vi "json is equal.vi"(8 "error in (no error)":errorcluster, 9 "json string B":string, 10 "json string A":string, 11 "TestCase in":refnum<class "TestCase.lvclass">) -> (0 "error out":errorcluster, 3 "TestCase out":refnum<class "TestCase.lvclass">)   [LabVIEW 2017]
uses:
  <vilib>/addons/_JKI Toolkits/VI Tester/TestCase.llb/TestCase.lvclass
  <vilib>/National Instruments/Variant Data Manipulation/Path API/Read Value at Path(String).vi
  <vilib>/National Instruments/Variant JSON API/Variant JSON API.lvlib
  <vilib>/National Instruments/Variant Data Manipulation/Variant Data Manipulation.lvlib
  <vilib>/Utility/Data Type/NI_Data Type.lvlib
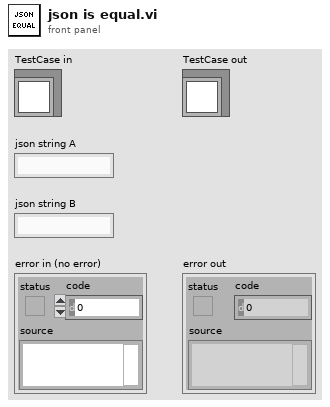
[diagram p1: front panel]
types:
  T1 = typedef "NI_Data Type.lvlib/Data Type.ctl" = enum8{"Invalid Type", "Void", "I8", "I16", "I32", "I64", "U8", "U16", "U32", "U64", "Single Float", "Double Float", "Extended Float", "Single Complex", "Double Complex", "Extended Complex", "Enum U8", "Enum U16", "Enum U32", "Enum U64", "Single Float With Unit", "Double Float With Unit", "Extended Float With Unit", "Single Complex with Unit", "Double Complex with Unit", "Extended Complex with Unit", "Boolean", "String", "Path", "Picture", "Tag", "Array", "Cluster", "Variant", "LV Variant", "Waveform", "Timestamp", "Digital Waveform", "Digital Data", "ExpressData", "Refnum", "External Data", "VI", "Poly VI", "LabVIEW Class Instance", "Fixed Point"}
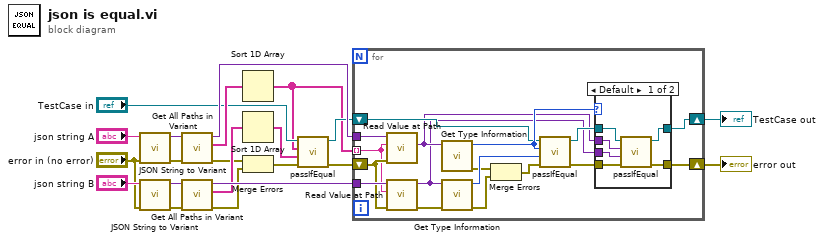
[diagram p0: block diagram]
diagram:
  n1 = call <vilib>:"JSON String to Variant.vi"("error in (no error)"="error in (no error)", "JSON String"="json string A") -> ("error out"=w1:errorcluster, "Variant out"=w19:variant)  [unwired: 8 in]
  n2 = call <vilib>:"JSON String to Variant.vi"("error in (no error)"="error in (no error)", "JSON String"="json string B") -> ("error out"=w17:errorcluster, "Variant out"=w18:variant)  [unwired: 8 in]
  n3 = call <vilib>:"Get All Paths in Variant.vi"("error in (no error)"=w1, "Variant in"=w19) -> ("error out"=w8:errorcluster, "Paths out"=w14:string[], "Variant out"=w16:variant)  [unwired: 7 in]
  n4 = call <vilib>:"Get All Paths in Variant.vi"("error in (no error)"=w17, "Variant in"=w18) -> ("error out"=w7:errorcluster, "Paths out"=w13:string[], "Variant out"=w15:variant)  [unwired: 7 in]
  n5 = Sort 1D Array(array=w14) -> (sorted array=w4:string[])
  n6 = Sort 1D Array(array=w13) -> (sorted array=w12:string[])
  n7 = Merge Errors(w8, w7) -> (w6:errorcluster)
  n8 = call-dynamic "passIfEqual.vi"("error in (no error)"=w6, "y"=w12, "x"=w4, "TestCase in"="TestCase in") -> ("error out"=w5:errorcluster, "TestCase out"=w11:refnum<class "TestCase.lvclass">)  [unwired: 6 in]
  n9 = for {
    tunnel: w16 -> [w38]
    tunnel: w15 -> [w37]
    tunnel: w4 -> [w22] mode=indexing
    shift-right: [w23] -> w3
    shift-left: w11 -> [w33]
    shift-right: [w24] -> w2
    shift-left: w5 -> [w29]
    n10 = call-poly <vilib>:"Read Value at Path.vi"("error in (no error)"=w29, "Path String"=w22, "Variant in"=w38) -> ("Element out"=w31:variant)  [unwired: 6 in, 2 out]
    n11 = call-poly <vilib>:"Read Value at Path.vi"("error in (no error)"=w29, "Path String"=w22, "Variant in"=w37) -> ("error out"=w36:errorcluster, "Variant out"=w30:variant)  [unwired: 6 in, 1 out]
    n12 = call <vilib>:"Get Type Information.vi"("Variant"=w31) -> ("error out"=w28:errorcluster, "Type"=w34:T1)  [unwired: 6 in, 3 out]
    n13 = call <vilib>:"Get Type Information.vi"("error in (no error)"=w36, "Variant"=w30) -> ("error out"=w27:errorcluster, "Type"=w35:T1)  [unwired: 5 in, 3 out]
    n14 = Merge Errors(w28, w27) -> (w26:errorcluster)
    n15 = call-dynamic "passIfEqual.vi"("error in (no error)"=w26, "y"=w35, "x"=w34, "TestCase in"=w33) -> ("error out"=w25:errorcluster, "TestCase out"=w32:refnum<class "TestCase.lvclass">)  [unwired: 6 in]
    n16 = case shown="Default" w34 {
      tunnel: w32 -> [w40 w46]
      tunnel: w31 -> [w44 _]
      tunnel: w30 -> [w43 _]
      tunnel: w25 -> [w42 w45]
      tunnel: [w41 w45] -> w24
      tunnel: [w39 w46] -> w23
      frame Default {
        n17 = call-dynamic "passIfEqual.vi"("error in (no error)"=w42, "y"=w43, "x"=w44, "TestCase in"=w40) -> ("error out"=w41:errorcluster, "TestCase out"=w39:refnum<class "TestCase.lvclass">)  [unwired: 6 in]
      }
      frame "Array", "Cluster" {
      }
    }
  }
  "error out" <- w2
  "TestCase out" <- w3
